vi "control_lasers_from_CSV_gui_demo.vi"() -> ()   [LabVIEW 2021]
uses:
  <vilib>/DAQmx/write.llb/DAQmx Write (Analog 1D DBL NChan 1Samp).vi
  <vilib>/DAQmx/create/channels.llb/DAQmx Create Channel (AO-Voltage-Basic).vi
  <vilib>/Utility/file.llb/Read Delimited Spreadsheet (DBL).vi
  <vilib>/DAQmx/configure/timing.llb/DAQmx Timing (Sample Clock).vi
  <vilib>/DAQmx/miscellaneous.llb/DAQmx Fill In Error Info.vi
  <vilib>/measure/NI_MABase.lvlib
panel:
  in  "Waveplate (set and forget)":dbl
  out "ETL3 Current":dbl(graph)
  out "Andor Output Logs":dbl(graph)
  in  "RUN":bool
  out "ETL2 Current":dbl(graph)
  in  "Y2":dbl
  in  "X2":dbl
  out "Camera Frames":dbl
  out "Lightsheet Angle":dbl(graph)
  out "Elapsed Time":dbl
  out "LS SweepPosition":dbl(graph)
  out "Power Output":dbl(graph)
  out "3-D Scans Completed":i32
  out "561 (Automated)":dbl
  out "Plane Scans":i32
  in  "TickLength":u32
  in  "Y1 (-10-10V)":dbl
  in  "X1 (-10-10V)":dbl
  in  "Blanking (0-10v)":dbl=10.0
  in  "514 (0-10v)":dbl
  in  "488 (0-10v)":dbl
  in  "445 (0-10v)":dbl
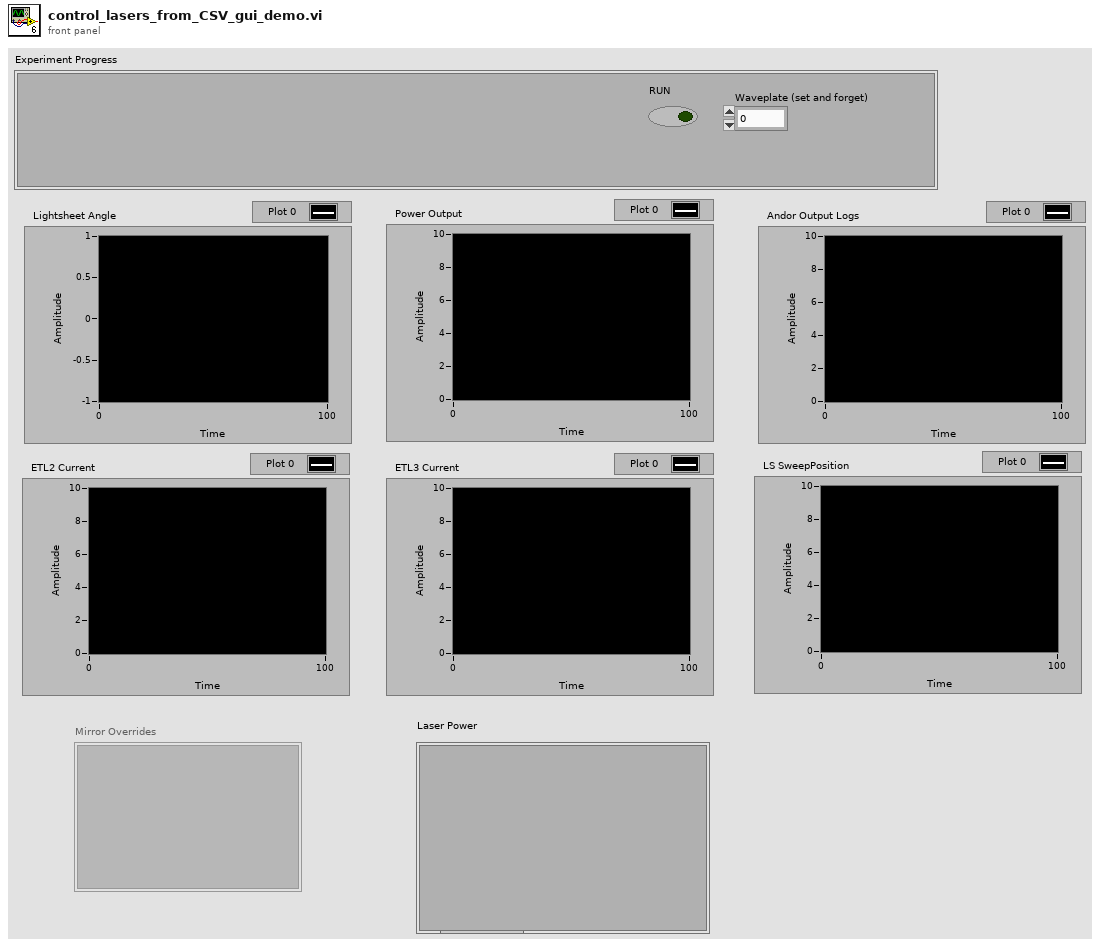
[diagram p1: front panel]
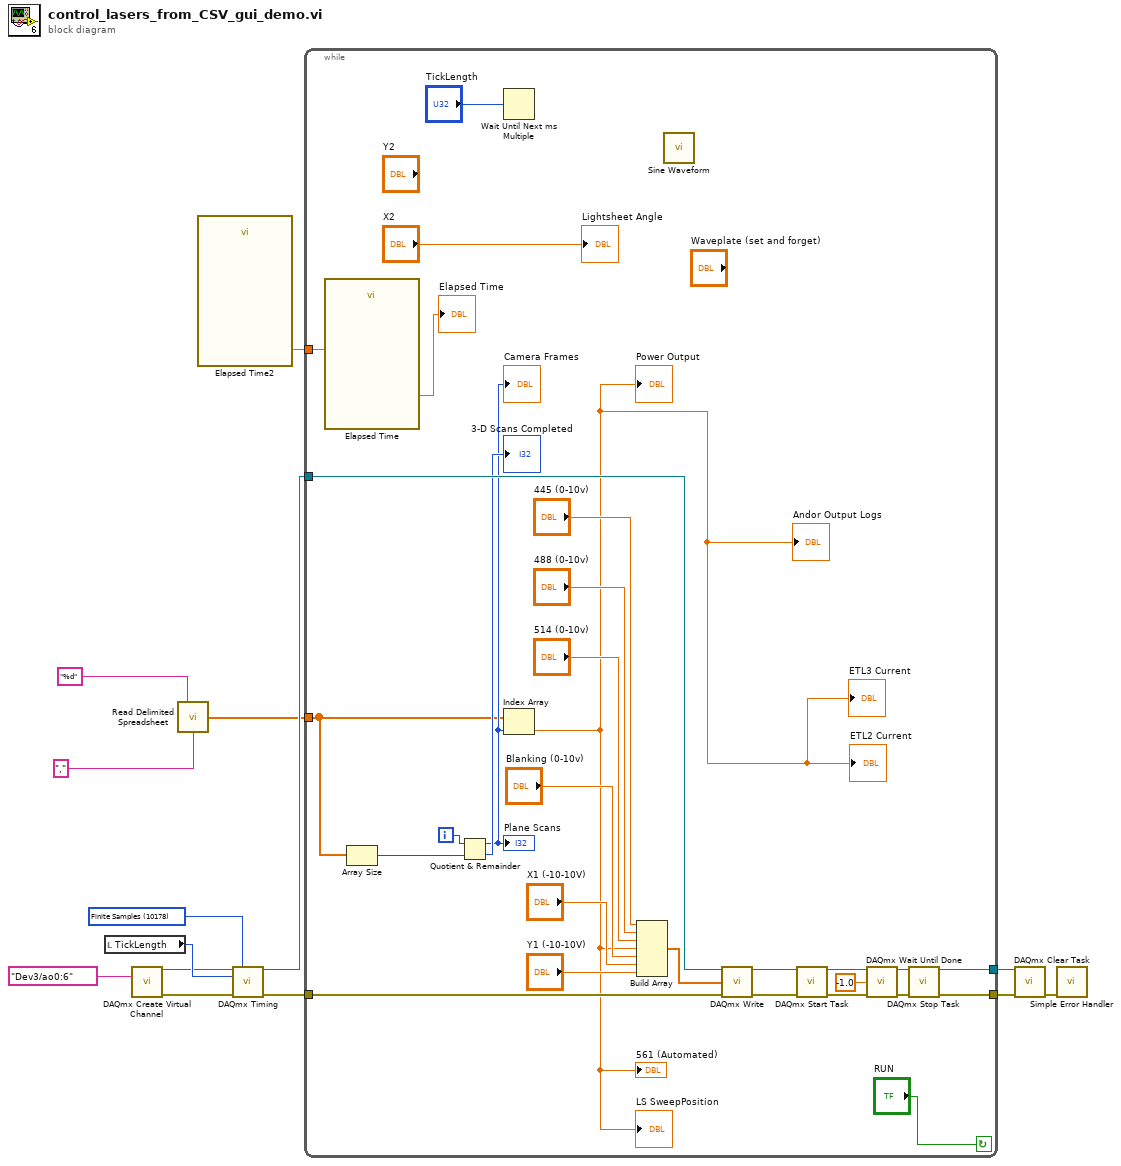
[diagram p0: block diagram]
diagram:
  w12 = 10178 items=["Finite Samples"=10178, "Continuous Samples"=10123, "Hardware Timed Single Point"=12522] ("sample mode")
  n1 = local read "TickLength"() -> (w11:u32)
  n2 = call-poly <vilib>:"DAQmx Create Virtual Channel.vi"("physical channels"=tag "Dev3/ao0:6") -> ("task out"=w8:refnum<k21>, "error out"=w7:errorcluster)  [unwired: 13 in]
  n3 = call-poly <vilib>:"Read Delimited Spreadsheet.vi"("format (%.3f)"="%d", "delimiter (\\t)"=",") -> ("first row"=w2:dbl[])  [unwired: 8 in, 5 out]
  n4 = call "Elapsed Time2"() -> ("Present (s)"=w1:dbl)  [unwired: 12 in, 7 out]
  n5 = call-poly <vilib>:"DAQmx Timing.vi"("task/channels in"=w8, "sample mode"=w12, "rate"=w11, "error in"=w7) -> ("task out"=w5:refnum<k21>, "error out"=w6:errorcluster)  [unwired: 10 in]
  n6 = while {
    tunnel: [w30] -> w10
    tunnel: [w31] -> w9
    tunnel: w6 -> [w26]
    tunnel: w5 -> [w25]
    tunnel: w2 -> [w17]
    tunnel: w1 -> [w21]
    i -> [w24]
    stop <- "RUN" continue-if-true
    n7 = call "Elapsed Time"("Set Start Time (s)"=w21) -> ("Elapsed Time (s)"=→"Elapsed Time":dbl)  [unwired: 11 in, 7 out]
    n8 = Array Size(array=w17) -> (size(s)=w23:i32)
    n9 = Quotient & Remainder(x=w24, y=w23) -> (x-y*floor(x/y)=w19:i32, floor(x/y)=→"3-D Scans Completed":i32)
    "Plane Scans" <- w19
    "Camera Frames" <- w19
    n10 = Wait Until Next ms Multiple(millisecond multiple="TickLength") -> ()  [unwired: 1 out]
    n11 = Index Array "Index Array"(array=w17, index=w19) -> (element=w15:dbl)
    "561 (Automated)" <- w15
    "LS SweepPosition" <- w15
    "Power Output" <- w15
    "ETL2 Current" <- w15
    "ETL3 Current" <- w15
    "Andor Output Logs" <- w15
    n12 = Build Array("445 (0-10v)", "488 (0-10v)", "514 (0-10v)", w15, "Blanking (0-10v)", "X1 (-10-10V)", "Y1 (-10-10V)") -> (w43:dbl[])
    n13 = call <vilib>:"Sine Waveform.vi"() -> ()  [unwired: 10 in, 2 out]
    n14 = call-poly <vilib>:"DAQmx Write.vi"("task/channels in"=w25, "data"=w43, "error in"=w26) -> ("task out"=w27:refnum<k21>, "error out"=w34:errorcluster)  [unwired: 10 in, 1 out]
    n15 = call <vilib>:"DAQmx Start Task.vi"("task/channels in"=w27, "error in"=w34) -> ("task out"=w28:refnum<k21>, "error out"=w33:errorcluster)  [unwired: 12 in]
    n16 = call <vilib>:"DAQmx Wait Until Done.vi"("task/channels in"=w28, "timeout (sec)"=-1.0, "error in"=w33) -> ("task out"=w29:refnum<k21>, "error out"=w32:errorcluster)  [unwired: 11 in]
    n17 = call <vilib>:"DAQmx Stop Task.vi"("task/channels in"=w29, "error in"=w32) -> ("task out"=w30:refnum<k21>, "error out"=w31:errorcluster)  [unwired: 12 in]
    "Lightsheet Angle" <- "X2"
  }
  n18 = call <vilib>:"DAQmx Clear Task.vi"("task in"=w10, "error in"=w9) -> ("error out"=w14:errorcluster)  [unwired: 13 in]
  n19 = call <vilib>:"Simple Error Handler.vi"("error in (no error)"=w14) -> ()  [unwired: 4 in, 5 out]
